vi "set_ref_clus_BGA244.vi"(6 "cluster_ref_BGA244":T1, 10 "purity":dbl, 11 "status":bool) -> ()   [LabVIEW 2019]
uses:
  cluster_ref_BGA244.ctl
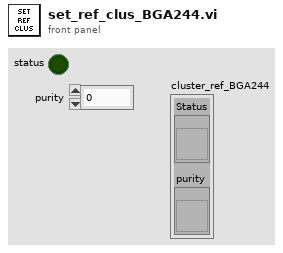
[diagram p1: front panel]
types:
  T1 = typedef "cluster_ref_BGA244.ctl" = cluster{"Status":refnum<vi>, "purity":refnum<vi>}
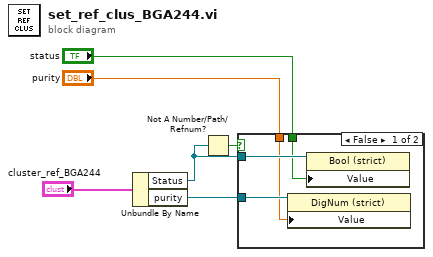
[diagram p0: block diagram]
diagram:
  n1 = Unbundle By Name("cluster_ref_BGA244") -> ("Status"=w4:refnum<vi>, "purity"=w5:refnum<vi>)
  n2 = Not A Number/Path/Refnum?(number/path/refnum=w4) -> (NaN/Path/Refnum?=w6:bool)
  n3 = case shown="False" w6 {
    tunnel: w5 -> [w10 _]
    tunnel: w4 -> [w9 _]
    tunnel: "status" -> [w8 _]
    tunnel: "purity" -> [w7 _]
    frame False {
      n4 = property class="DigNum (strict)"(reference=w10, "Value"=w7) -> ()  [unwired: 1 in, 2 out]
      n5 = property class="Bool (strict)"(reference=w9, "Value"=w8) -> ()  [unwired: 1 in, 2 out]
    }
    frame True {
    }
  }
